vi "Dialog Tester.vi"() -> ()   [LabVIEW 2021]
doc: "<b>TEST VI</b> meant to check status of all standard or custom popups so that you can see how they are displayed"
uses:
  Custom/Custom - Input (DBL)/Custom - Input (DBL).lvclass
  Custom/Custom - Input (I32)/Custom - Input (I32).lvclass
  Custom/Custom - Input (String)/Custom - Input (String).lvclass
  Custom/Custom - One Button/Custom - One Button.lvclass
  Custom/Custom - Timeout/Custom - Timeout.lvclass
  Custom/Custom - Timeout One Button/Custom - Timeout One Button.lvclass
  Custom/Custom - Timeout Two Button/Custom - Timeout Two Button.lvclass
  Custom/Custom - Two Button/Custom - Two Button.lvclass
  Standard/Input (DBL)/Input (DBL).lvclass
  Graphics.ctl
  Pop-Up.lvlib
  Standard/Input (I32)/Input (I32).lvclass
  Standard/Input (String)/Input (String).lvclass
  Standard/One Button/One Button.lvclass
  Standard/Timeout/Timeout.lvclass
  Standard/Timeout One Button/Timeout One Button.lvclass
  Standard/Timeout Two Button/Timeout Two Button.lvclass
  Standard/Two Button/Two Button.lvclass
  Theme/Theme.lvclass
panel:
  in  "Background?":bool
  out "iteration":i32
  in  "Pop Up Type":enum16{"Custom", "Standard"}(ring)
  in  "Error In":errorcluster
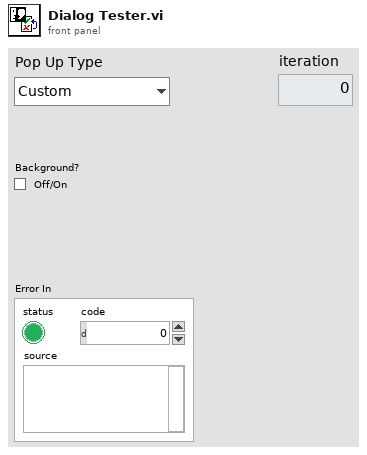
[diagram p1: front panel]
types:
  T1 = typedef "Pop-Up.lvlib/Graphics.ctl" = string
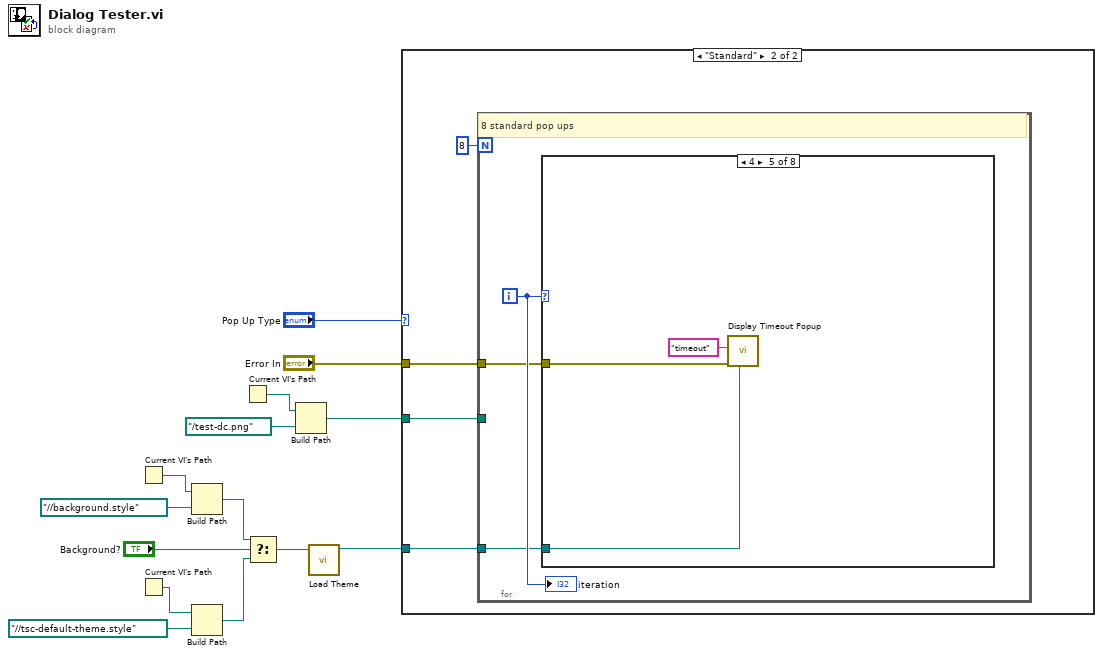
[diagram p0: block diagram]
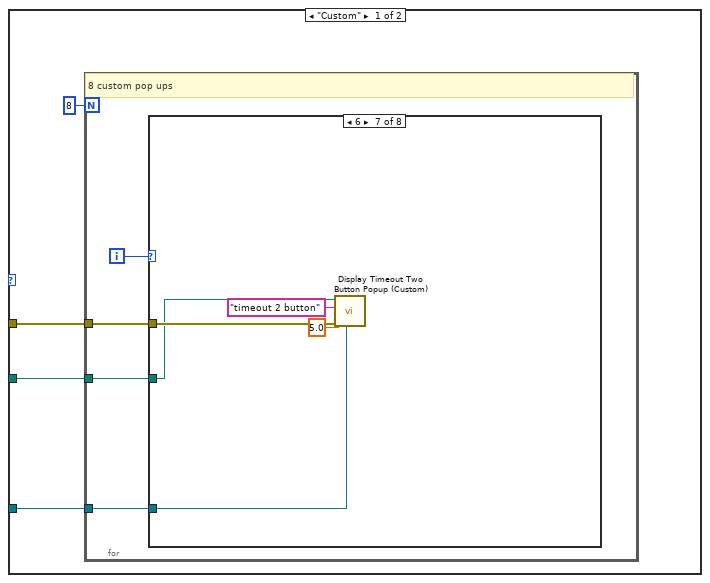
[diagram p2: hidden frame]
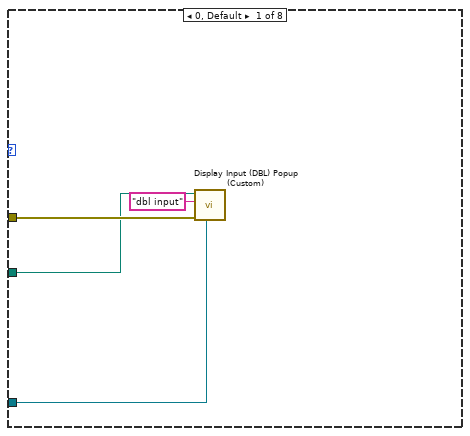
[diagram p3: hidden frame]
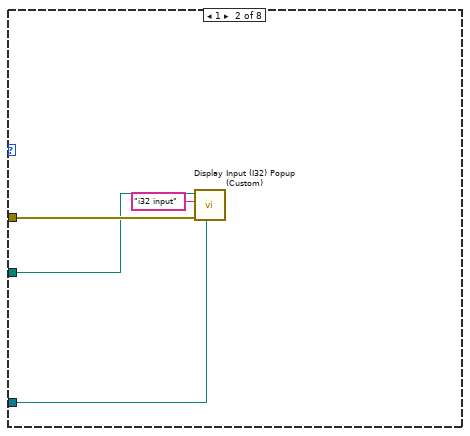
[diagram p4: hidden frame]
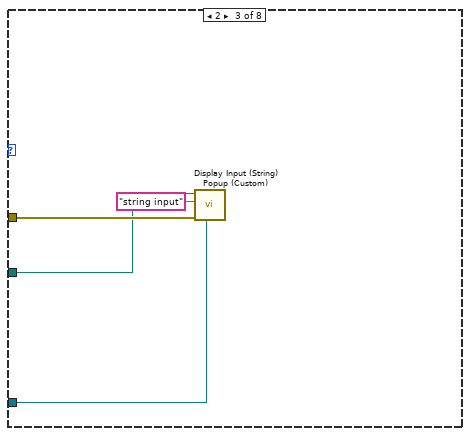
[diagram p5: hidden frame]
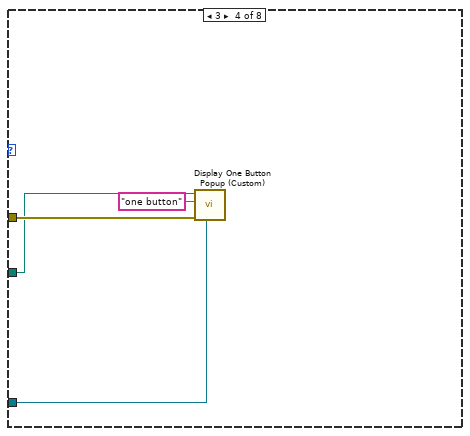
[diagram p6: hidden frame]
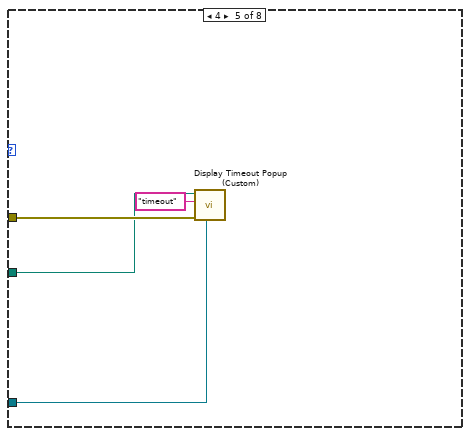
[diagram p7: hidden frame]
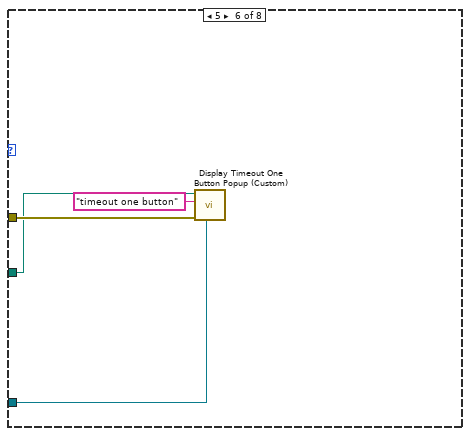
[diagram p8: hidden frame]
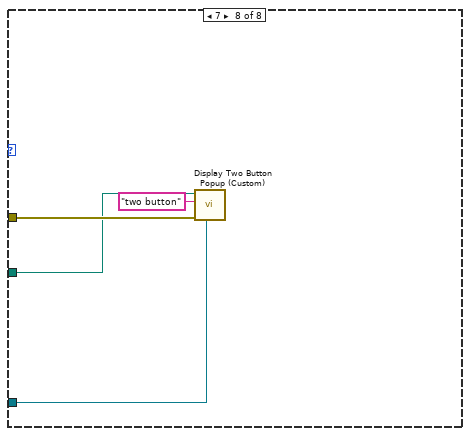
[diagram p9: hidden frame]
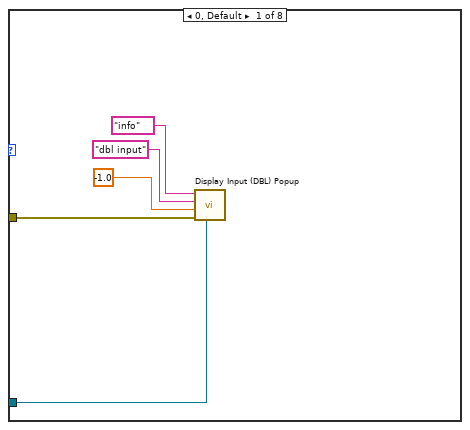
[diagram p10: hidden frame]
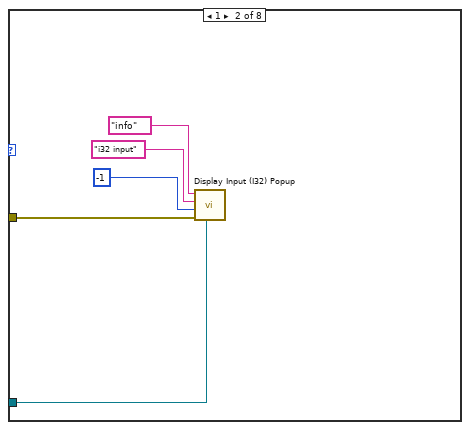
[diagram p11: hidden frame]
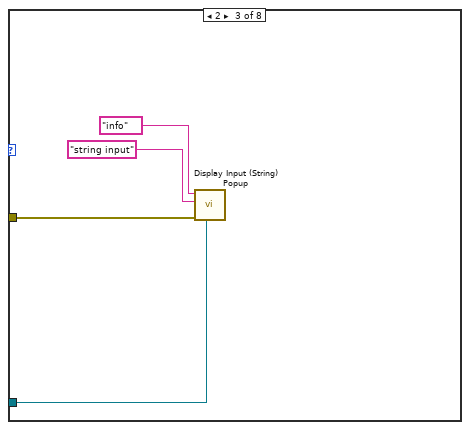
[diagram p12: hidden frame]
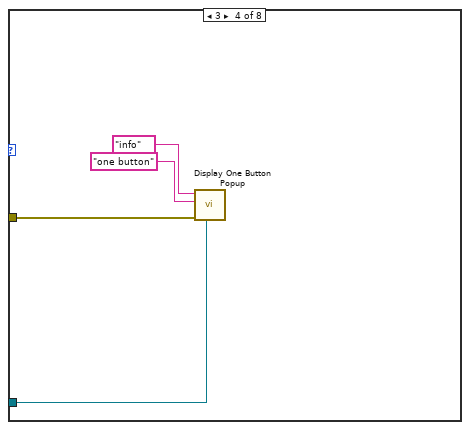
[diagram p13: hidden frame]
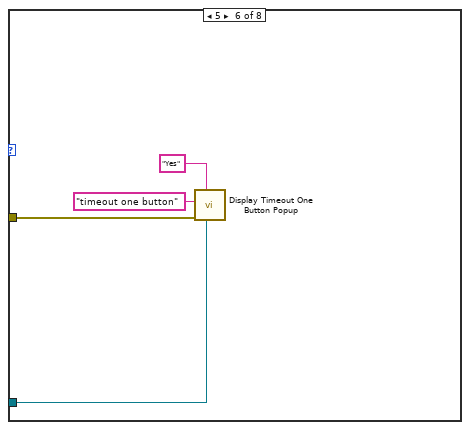
[diagram p14: hidden frame]
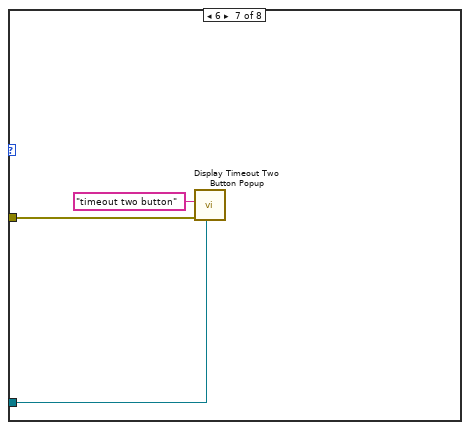
[diagram p15: hidden frame]
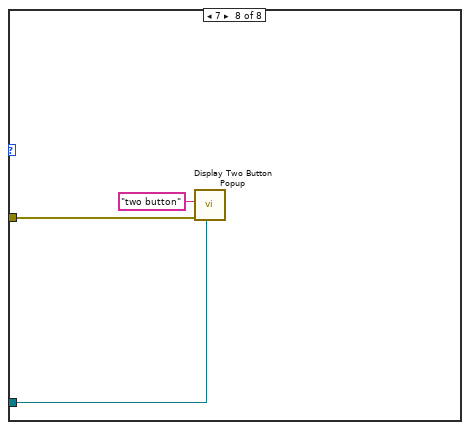
[diagram p16: hidden frame]
diagram:
  n1 = Current VI's Path() -> (path=w8:path)
  n2 = Current VI's Path() -> (path=w3:path)
  n3 = Build Path(base path=w8, name or relative path=path "../../background.style") -> (appended path=w7:path)
  n4 = Build Path(base path=w3, name or relative path=path "../../tsc-default-theme.style") -> (appended path=w4:path)
  n5 = Current VI's Path() -> (path=w14:path)
  n6 = Select(t=w7, s="Background?", f=w4) -> (s? t:f=w6:path)
  n7 = Build Path(base path=w14, name or relative path=path "../test-dc.png") -> (appended path=w12:path)
  n8 = call "Load Theme.vi"("File Path"=w6) -> ("Theme"=w1:refnum<class "Theme.lvclass">)  [unwired: 9 in, 1 out]
  n9 = case shown="\"Standard\"" "Pop Up Type" {
    tunnel: w12 -> [w17 w58]
    tunnel: "Error In" -> [w16 w57]
    tunnel: w1 -> [w15 w56]
    frame "Custom" {
      n10 = for {
        N: 8 -> [_]
        tunnel: w17 -> [w21]
        tunnel: w16 -> [w20]
        tunnel: w15 -> [w19]
        i -> [w22]
        # "8 custom pop ups"
        n11 = case shown="6" w22 {
          tunnel: w21 -> [w25 w29 w33 w37 w41 w45 w50 w54]
          tunnel: w20 -> [w26 w30 w34 w38 w42 w46 w51 w55]
          tunnel: w19 -> [w23 w27 w31 w35 w39 w43 w47 w52]
          frame 0, Default {
            n12 = call "Display Input (DBL) Popup (Custom).vi"("Theme"=w23, "Error In"=w26, "Message"="dbl input", "Graphic"=w25) -> ()  [unwired: 6 in, 2 out]
          }
          frame 1 {
            n13 = call "Display Input (I32) Popup (Custom).vi"("Theme"=w27, "Error In"=w30, "Message"="i32 input", "Graphic"=w29) -> ()  [unwired: 6 in, 2 out]
          }
          frame 2 {
            n14 = call "Display Input (String) Popup (Custom).vi"("Theme"=w31, "Error In"=w34, "Message"="string input", "Graphic"=w33) -> ()  [unwired: 6 in, 2 out]
          }
          frame 3 {
            n15 = call "Display One Button Popup (Custom).vi"("Theme"=w35, "Error In"=w38, "Message"="one button", "Graphic"=w37) -> ()  [unwired: 7 in, 1 out]
          }
          frame 4 {
            n16 = call "Display Timeout Popup (Custom).vi"("Theme"=w39, "Error In"=w42, "Message"="timeout", "Graphic"=w41) -> ()  [unwired: 6 in, 2 out]
          }
          frame 5 {
            n17 = call "Display Timeout One Button Popup (Custom).vi"("Theme"=w43, "Error In"=w46, "Message"="timeout one button", "Graphic"=w45) -> ()  [unwired: 6 in, 2 out]
          }
          frame 6 {
            n18 = call "Display Timeout Two Button Popup (Custom).vi"("Theme"=w47, "Error In"=w51, "Timeout (s)"=5.0, "Message"="timeout 2 button", "Graphic"=w50) -> ()  [unwired: 4 in, 3 out]
          }
          frame 7 {
            n19 = call "Display Two Button Popup (Custom).vi"("Theme"=w52, "Error In"=w55, "Message"="two button", "Graphic"=w54) -> ()  [unwired: 6 in, 2 out]
          }
        }
      }
    }
    frame "Standard" {
      n20 = for {
        N: 8 -> [_]
        tunnel: w58 -> [_]
        tunnel: w57 -> [w61]
        tunnel: w56 -> [w60]
        i -> [w62]
        # "8 standard pop ups"
        n21 = case shown="4" w62 {
          tunnel: w61 -> [w67 w72 w76 w80 w83 w87 w90 w93]
          tunnel: w60 -> [w63 w68 w73 w77 w81 w84 w88 w91]
          frame 0, Default {
            n22 = call "Display Input (DBL) Popup.vi"("Theme"=w63, "error in"=w67, "Default Input"=-1.0, "Message"="dbl input", "Graphic"=T1 "info") -> ()  [unwired: 5 in, 2 out]
          }
          frame 1 {
            n23 = call "Display Input (I32) Popup.vi"("Theme"=w68, "error in"=w72, "Default Input"=-1, "Message"="i32 input", "Graphic"=T1 "info") -> ()  [unwired: 5 in, 2 out]
          }
          frame 2 {
            n24 = call "Display Input (String) Popup.vi"("Theme"=w73, "error in"=w76, "Message"="string input", "Graphic"=T1 "info") -> ()  [unwired: 6 in, 2 out]
          }
          frame 3 {
            n25 = call "Display One Button Popup.vi"("Theme"=w77, "error in"=w80, "Message"="one button", "Graphic"=T1 "info") -> ()  [unwired: 7 in, 1 out]
          }
          frame 4 {
            n26 = call "Display Timeout Popup.vi"("Theme"=w81, "error in"=w83, "Message"="timeout") -> ()  [unwired: 7 in, 2 out]
          }
          frame 5 {
            n27 = call "Display Timeout One Button Popup.vi"("Theme"=w84, "Button Text"="Yes", "error in"=w87, "Message"="timeout one button") -> ()  [unwired: 6 in, 2 out]
          }
          frame 6 {
            n28 = call "Display Timeout Two Button Popup.vi"("Theme"=w88, "error in"=w90, "Message"="timeout two button") -> ()  [unwired: 6 in, 3 out]
          }
          frame 7 {
            n29 = call "Display Two Button Popup.vi"("Theme"=w91, "error in"=w93, "Message"="two button") -> ()  [unwired: 7 in, 2 out]
          }
        }
        "iteration" <- w62
      }
    }
  }
